vi "Open Sensors and Actuators.vi"   [LabVIEW 2014]
uses:
  <vilib>/Rock Robotics/SystemInterfaces/DIO/FPGA_DIOPWMChannel.ctl
  <vilib>/Rock Robotics/SystemInterfaces/AI/FPGA_AIChannel.ctl
  <vilib>/Rock Robotics/WPI/Joystick/WPI_JoystickDeviceEnum.ctl
  <vilib>/Rock Robotics/SystemInterfaces/DIO/FPGA_DIOChannel.ctl
  <vilib>/Rock Robotics/WPI/MotorControl/WPI_MotorControlOpen Talon.vi
  <vilib>/Rock Robotics/WPI/MotorControl/WPI_MotorControlOpen Victor.vi
  <vilib>/Rock Robotics/WPI/Counter/WPI_CounterDigitalInputToDigitalSource.vi
  <vilib>/Rock Robotics/WPI/Counter/WPI_CounterOpen Gear Tooth Sensor Mode.vi
  Global RefNums.vi
types:
  T1 = typedef "FPGA_DIOChannel.ctl" = enum8{"DIO 0", "DIO 1", "DIO 2", "DIO 3", "DIO 4", "DIO 5", "DIO 6", "DIO 7", "DIO 8", "DIO 9", "DIO MXP 0", "DIO MXP 1", "DIO MXP 2", "DIO MXP 3", "DIO MXP 4", "DIO MXP 5", "DIO MXP 6", "DIO MXP 7", "DIO MXP 8", "DIO MXP 9", "DIO MXP 10", "DIO MXP 11", "DIO MXP 12", "DIO MXP 13", "DIO MXP 14", "DIO MXP 15", "Invalid"}
  T2 = typedef "WPI_JoystickDeviceEnum.ctl" = enum16{"USB 0", "USB 1", "USB 2", "USB 3", "USB 4", "USB 5"}
  T3 = typedef "FPGA_AIChannel.ctl" = enum8{"AI 0", "AI 1", "AI 2", "AI 3", "AI MXP 0", "AI MXP 1", "AI MXP 2", "AI MXP 3", "Invalid"}
  T4 = typedef "FPGA_DIOPWMChannel.ctl" = enum8{"PWM 0", "PWM 1", "PWM 2", "PWM 3", "PWM 4", "PWM 5", "PWM 6", "PWM 7", "PWM 8", "PWM 9", "PWM MXP 0", "PWM MXP 1", "PWM MXP 2", "PWM MXP 3", "PWM MXP 4", "PWM MXP 5", "PWM MXP 6", "PWM MXP 7", "PWM MXP 8", "PWM MXP 9", "Invalid"}
  T5 = typedef "WPI_MotorControlDeviceRef.ctl" = cluster{"DeviceStatus":errorcluster, "Type":T6, "PWM":cluster{"Controller":T7, "PWM Channel":T4, "DeadBand":T8}, "CAN":cluster{"Device Number":u8, "Control Mode":T9, "Semaphore":T10, "Max Vout":dbl, "TalonSRX Control Mode":T11}, "Invert":bool, "TransformRef":T12, "InvTransformRef":T12}
  T6 = typedef "WPI_MotorControlType.ctl" = enum16{"PWM", "CAN", "CANTalonSRX"}
  T7 = typedef "FPGA_TypedefDigitalModule.ctl" = enum16{"Controller 1"}
  T8 = typedef "WPI_PWMDeadband.ctl" = cluster{"Name":string, "maxPositivePwm":i32, "minPositivePwm":i32, "centerPwm":i32, "maxNegativePwm":i32, "minNegativePwm":i32, "angularRange":u16}
  T9 = typedef "WPI_CANJaguar_ControlMode.ctl" = enum8{"Percent VBus", "Current", "Speed", "Position", "Voltage"}
  T10 = typedef "Semaphore RefNum" = refnum<k1>
  T11 = typedef "WPI_CANTalonSRX_APIControlMode.ctl" = enum8{"Percent VBus", "Speed", "Position", "Slave", "Unchanged / Invalid"}
  T12 = typedef "WPI_PWMTransform_ConPane.ctl" = refnum<vi>
  T13 = typedef "WPI_JoystickDevRef.ctl" = cluster{"Device":T2}
  T14 = typedef "WPI_AnalogChannelDevRef.ctl" = cluster{"DevStatus":errorcluster, "Controller":T15, "Analog Channel":T3}
  T15 = typedef "FPGA_TypedefAnalogModule.ctl" = enum16{"Controller 1"}
  T16 = typedef "WPI_DigitalInputDevRef.ctl" = cluster{"DevStatus":errorcluster, "DIO Channel":T1, "Controller":T7}
  T17 = typedef "FPGA_CounterEncoderSourceConvertionLVSourceType.ctl" = cluster{"DevStatus":errorcluster, "AnalogTriggerMode?":bool, "DigitalMode":cluster{"Controller":T7, "DIO Channel":T18}, "AnalogTriggerMode":cluster{"AnalogTriggerIndex":T19, "OutputType":T20}}
  T18 = typedef "FPGA_DIODigitalSourceChannel.ctl" = enum8{"DIO 0", "DIO 1", "DIO 2", "DIO 3", "DIO 4", "DIO 5", "DIO 6", "DIO 7", "DIO 8", "DIO 9", "DIO MXP 0", "DIO MXP 1", "DIO MXP 2", "DIO MXP 3", "DIO MXP 4", "DIO MXP 5", "DIO MXP 6", "DIO MXP 7", "DIO MXP 8", "DIO MXP 9", "DIO MXP 10", "DIO MXP 11", "DIO MXP 12", "DIO MXP 13", "DIO MXP 14", "DIO MXP 15", "Disabled"}
  T19 = typedef "FPGA_AnalogTriggerIndex.ctl" = enum8{"Trig 0", "Trig 1", "Trig 2", "Trig 3", "Trig 4", "Trig 5", "Trig 6", "Trig 7", "Invalid"}
  T20 = typedef "FPGA_AnalogTriggerOutType.ctl" = enum16{"InWindow", "TriggerState", "Rising", "Falling"}
  T21 = typedef "WPI_CounterDevRef.ctl" = cluster{"DevStatus":errorcluster, "CntIndex":T22}
  T22 = typedef "FPGA_CounterCtrSystemIndex.ctl" = enum8{"Ctr 0", "Ctr 1", "Ctr 2", "Ctr 3", "Ctr 4", "Ctr 5", "Ctr 6", "Ctr 7", "Invalid"}
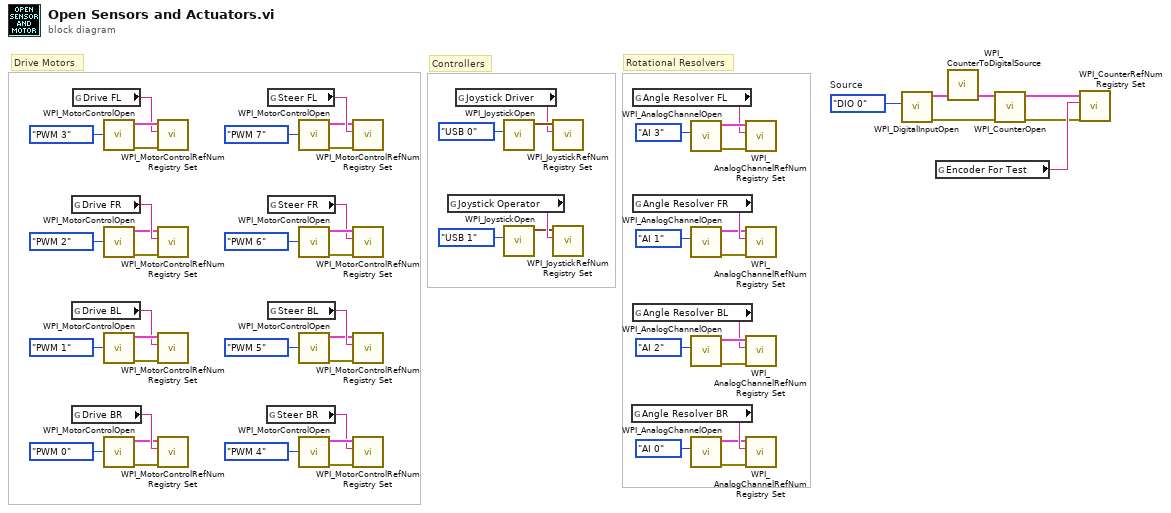
[diagram p0: block diagram]
diagram:
  w6 = FPGA_DIOChannel."DIO 0"  # Source
  # "Drive Motors"
  # "Controllers"
  # "Rotational Resolvers"
  n1 = global read "Global RefNums.vi" "Drive FR"() -> (w53:string)
  n2 = global read "Global RefNums.vi" "Drive BL"() -> (w48:string)
  n3 = global read "Global RefNums.vi" "Drive BR"() -> (w45:string)
  n4 = global read "Global RefNums.vi" "Drive FL"() -> (w56:string)
  n5 = call-poly <vilib>:"WPI_MotorControlOpen.vi"("PWM Channel"=FPGA_DIOPWMChannel."PWM 3") -> ("error out"=w57:errorcluster, "MotorControlDeviceRef"=w58:T5)  [unwired: 9 in]
  n6 = call-poly <vilib>:"WPI_MotorControlOpen.vi"("PWM Channel"=FPGA_DIOPWMChannel."PWM 2") -> ("error out"=w52:errorcluster, "MotorControlDeviceRef"=w51:T5)  [unwired: 9 in]
  n7 = call-poly <vilib>:"WPI_MotorControlOpen.vi"("PWM Channel"=FPGA_DIOPWMChannel."PWM 1") -> ("error out"=w49:errorcluster, "MotorControlDeviceRef"=w50:T5)  [unwired: 9 in]
  n8 = call-poly <vilib>:"WPI_MotorControlOpen.vi"("PWM Channel"=FPGA_DIOPWMChannel."PWM 0") -> ("error out"=w44:errorcluster, "MotorControlDeviceRef"=w43:T5)  [unwired: 9 in]
  n9 = call <vilib>:"WPI_MotorControlRefNum Registry Set.vi"("error in (no error)"=w57, "refnum name"=w56, "MotorControlDevRef"=w58) -> ()  [unwired: 7 in, 2 out]
  n10 = call <vilib>:"WPI_MotorControlRefNum Registry Set.vi"("error in (no error)"=w52, "refnum name"=w53, "MotorControlDevRef"=w51) -> ()  [unwired: 7 in, 2 out]
  n11 = call <vilib>:"WPI_MotorControlRefNum Registry Set.vi"("error in (no error)"=w49, "refnum name"=w48, "MotorControlDevRef"=w50) -> ()  [unwired: 7 in, 2 out]
  n12 = call <vilib>:"WPI_MotorControlRefNum Registry Set.vi"("error in (no error)"=w44, "refnum name"=w45, "MotorControlDevRef"=w43) -> ()  [unwired: 7 in, 2 out]
  n13 = global read "Global RefNums.vi" "Steer BR"() -> (w40:string)
  n14 = global read "Global RefNums.vi" "Steer FL"() -> (w29:string)
  n15 = global read "Global RefNums.vi" "Steer FR"() -> (w32:string)
  n16 = global read "Global RefNums.vi" "Steer BL"() -> (w37:string)
  n17 = call-poly <vilib>:"WPI_MotorControlOpen.vi"("PWM Channel"=FPGA_DIOPWMChannel."PWM 7") -> ("error out"=w28:errorcluster, "MotorControlDeviceRef"=w27:T5)  [unwired: 9 in]
  n18 = call-poly <vilib>:"WPI_MotorControlOpen.vi"("PWM Channel"=FPGA_DIOPWMChannel."PWM 6") -> ("error out"=w33:errorcluster, "MotorControlDeviceRef"=w34:T5)  [unwired: 9 in]
  n19 = call-poly <vilib>:"WPI_MotorControlOpen.vi"("PWM Channel"=FPGA_DIOPWMChannel."PWM 5") -> ("error out"=w36:errorcluster, "MotorControlDeviceRef"=w35:T5)  [unwired: 9 in]
  n20 = call-poly <vilib>:"WPI_MotorControlOpen.vi"("PWM Channel"=FPGA_DIOPWMChannel."PWM 4") -> ("error out"=w41:errorcluster, "MotorControlDeviceRef"=w42:T5)  [unwired: 9 in]
  n21 = call <vilib>:"WPI_MotorControlRefNum Registry Set.vi"("error in (no error)"=w28, "refnum name"=w29, "MotorControlDevRef"=w27) -> ()  [unwired: 7 in, 2 out]
  n22 = call <vilib>:"WPI_MotorControlRefNum Registry Set.vi"("error in (no error)"=w33, "refnum name"=w32, "MotorControlDevRef"=w34) -> ()  [unwired: 7 in, 2 out]
  n23 = call <vilib>:"WPI_MotorControlRefNum Registry Set.vi"("error in (no error)"=w36, "refnum name"=w37, "MotorControlDevRef"=w35) -> ()  [unwired: 7 in, 2 out]
  n24 = call <vilib>:"WPI_MotorControlRefNum Registry Set.vi"("error in (no error)"=w41, "refnum name"=w40, "MotorControlDevRef"=w42) -> ()  [unwired: 7 in, 2 out]
  n25 = global read "Global RefNums.vi" "Joystick Operator"() -> (w25:string)
  n26 = global read "Global RefNums.vi" "Joystick Driver"() -> (w26:string)
  n27 = call <vilib>:"WPI_JoystickOpen.vi"("JoystickDevice"=WPI_JoystickDeviceEnum."USB 0") -> ("JoystickDevRef"=w59:T13)  [unwired: 10 in]
  n28 = call <vilib>:"WPI_JoystickOpen.vi"("JoystickDevice"=WPI_JoystickDeviceEnum."USB 1") -> ("JoystickDevRef"=w24:T13)  [unwired: 10 in]
  n29 = call <vilib>:"WPI_JoystickRefNum Registry Set.vi"("refnum name"=w26, "JoystickDevRef"=w59) -> ()  [unwired: 8 in, 2 out]
  n30 = call <vilib>:"WPI_JoystickRefNum Registry Set.vi"("refnum name"=w25, "JoystickDevRef"=w24) -> ()  [unwired: 8 in, 2 out]
  n31 = global read "Global RefNums.vi" "Angle Resolver BR"() -> (w12:string)
  n32 = global read "Global RefNums.vi" "Angle Resolver FL"() -> (w23:string)
  n33 = global read "Global RefNums.vi" "Angle Resolver FR"() -> (w20:string)
  n34 = global read "Global RefNums.vi" "Angle Resolver BL"() -> (w15:string)
  n35 = call <vilib>:"WPI_AnalogChannelOpen.vi"("Analog Channel"=FPGA_AIChannel."AI 3") -> ("error out"=w61:errorcluster, "AIDeviceRef"=w60:T14)  [unwired: 9 in]
  n36 = call <vilib>:"WPI_AnalogChannelOpen.vi"("Analog Channel"=FPGA_AIChannel."AI 1") -> ("error out"=w18:errorcluster, "AIDeviceRef"=w19:T14)  [unwired: 9 in]
  n37 = call <vilib>:"WPI_AnalogChannelOpen.vi"("Analog Channel"=FPGA_AIChannel."AI 2") -> ("error out"=w17:errorcluster, "AIDeviceRef"=w16:T14)  [unwired: 9 in]
  n38 = call <vilib>:"WPI_AnalogChannelOpen.vi"("Analog Channel"=FPGA_AIChannel."AI 0") -> ("error out"=w10:errorcluster, "AIDeviceRef"=w11:T14)  [unwired: 9 in]
  n39 = call <vilib>:"WPI_AnalogChannelRefNum Registry Set.vi"("error in (no error)"=w61, "refnum name"=w23, "AIDeviceRef"=w60) -> ()  [unwired: 7 in, 2 out]
  n40 = call <vilib>:"WPI_AnalogChannelRefNum Registry Set.vi"("error in (no error)"=w18, "refnum name"=w20, "AIDeviceRef"=w19) -> ()  [unwired: 7 in, 2 out]
  n41 = call <vilib>:"WPI_AnalogChannelRefNum Registry Set.vi"("error in (no error)"=w17, "refnum name"=w15, "AIDeviceRef"=w16) -> ()  [unwired: 7 in, 2 out]
  n42 = call <vilib>:"WPI_AnalogChannelRefNum Registry Set.vi"("error in (no error)"=w10, "refnum name"=w12, "AIDeviceRef"=w11) -> ()  [unwired: 7 in, 2 out]
  n43 = call <vilib>:"WPI_DigitalInputOpen.vi"("DIO Channel"=w6) -> ("error out"=w1:errorcluster, "DigitalInputDevRef"=w5:T16)  [unwired: 2 in, 7 out]
  n44 = global read "Global RefNums.vi" "Encoder For Test"() -> (w3:string)
  n45 = call-poly <vilib>:"WPI_CounterToDigitalSource.vi"("DigitalInputDevRef"=w5) -> ("Digital Source"=w7:T17)  [unwired: 6 out]
  n46 = call-poly <vilib>:"WPI_CounterOpen.vi"("error in (no error)"=w1, "Source"=w7) -> ("error out"=w2:errorcluster, "CounterDevRef"=w4:T21)  [unwired: 5 in, 3 out]
  n47 = call <vilib>:"WPI_CounterRefNum Registry Set.vi"("error in (no error)"=w2, "refnum name"=w3, "CounterDevRef"=w4) -> ()  [unwired: 7 in, 2 out]
